vi "pid.calculate_backward_euler.vi"(6 "sampling_time (s)":dbl, 9 "Td":dbl, 10 "Ti":dbl, 11 "Kc":dbl) -> (2 "a1...an":dbl[](array[numeric]), 3 "b0...bn":dbl[](array[numeric]))   [LabVIEW 2015, in "discrete_control_systems.lvlib"]
doc: "Calculates the gains for a discrete difference equation from the PID controller parameters using the backward euler discretization method.\n\nThe implemented controller has the following equation in the LaPlace domain, where U(s) is the controller output:\n\nU(s) = Kc * ( 1 + 1/(Ti*s) + Td*s )"
uses:
  discrete_control_systems.lvlib
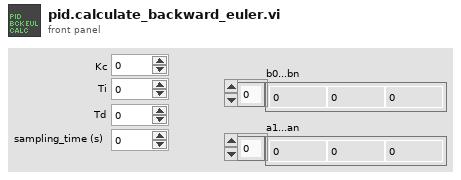
[diagram p1: front panel]
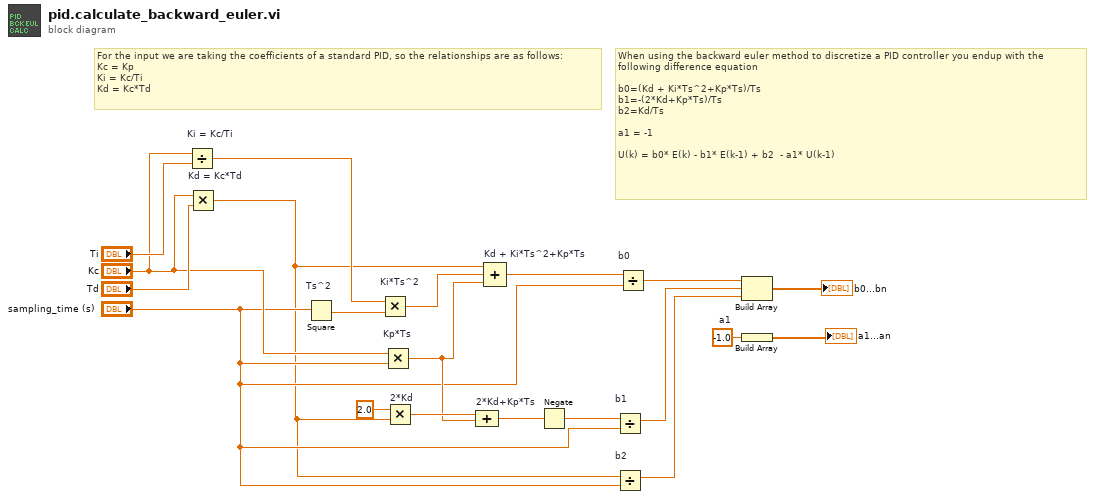
[diagram p0: block diagram]
diagram:
  w4 = -1.0  # a1
  # "For the input we are taking the coefficients of a standard PID, so the relationships are as follows:\nKc = Kp\nKi = Kc/Ti\nKd = Kc*Td"
  # "When using the backward euler method to discretize a PID controller you endup with the\nfollowing difference equation\n\nb0=(Kd + Ki*Ts^2+Kp*Ts)/Ts\nb1=-(2*Kd+Kp*Ts)/Ts\nb2=Kd/Ts\n\na1 = -1\n\nU(k) = b0* E(k) - b1* E(k-1) + b2  - a1* U(k-1)"
  n1 = Divide "Ki = Kc/Ti"(x="Kc", y="Ti") -> (x/y=w17:dbl)
  n2 = Multiply "Kd = Kc*Td"(x="Kc", y="Td") -> (x*y=w1:dbl)
  n3 = Square "Ts^2"(x="sampling_time (s)") -> (x^2=w18:dbl)
  n4 = Multiply "Ki*Ts^2"(x=w17, y=w18) -> (x*y=w15:dbl)
  n5 = Multiply "Kp*Ts"(x="Kc", y="sampling_time (s)") -> (x*y=w9:dbl)
  n6 = Multiply "2*Kd"(x=2.0, y=w1) -> (x*y=w13:dbl)
  n7 = Compound Arithmetic op=ADD "2*Kd+Kp*Ts"(w13, w9) -> (w11:dbl)
  n8 = Compound Arithmetic op=ADD "Kd + Ki*Ts^2+Kp*Ts"(w1, w15, w9) -> (w12:dbl)
  n9 = Negate(x=w11) -> (-x=w10:dbl)
  n10 = Divide "b1"(x=w10, y="sampling_time (s)") -> (x/y=w6:dbl)
  n11 = Divide "b2"(x=w1, y="sampling_time (s)") -> (x/y=w5:dbl)
  n12 = Divide "b0"(x=w12, y="sampling_time (s)") -> (x/y=w7:dbl)
  n13 = Build Array(w7, w6, w5) -> (→"b0...bn":dbl[])
  n14 = Build Array(w4) -> (→"a1...an":dbl[])
